vi "Destroy DataQ.vi"(6 "QueueName String (optional, otherwise \"\")":variant, 8 "error in (no error)":errorcluster, 9 "Select":T1, 10 "TaskName":string, 11 "DataQueues in":refnum<class "DataQueues.lvclass">) -> (0 "error out":errorcluster, 2 "TaskName out":string, 3 "DataQueues out":refnum<class "DataQueues.lvclass">)   [LabVIEW 2017, in "DataQueues.lvclass"]
doc: "Developed by Kevin Thompson\nkevin@thompsonengineering.net\n\nCopyright 2018-2020\nThompson Engineering, LLC"
uses:
  DataQueues.lvclass
  DataTypes/DataQ SelectType--enum.ctl
  DataQueues.lvclass/DataQueues.ctl
  DataTypes/DataQ Ref DictNode--cluster.ctl
  DataTypes/Analog DataSet SingleRow--QRef.ctl
  DataTypes/Analog DataSet SingleRow--cluster.ctl
  DataTypes/Analog DataSet MultiRow--QRef.ctl
  DataTypes/Analog DataSet MultiRow--cluster.ctl
  DataTypes/Analog DataSet MultiRow & ChanNames--QRef.ctl
  DataTypes/Analog DataSet MultiRow & ChanNames--cluster.ctl
  Accessors/Get QueueNames.vi
  Accessors/Get DataQ Dict.vi
  Accessors/Set QueueNames.vi
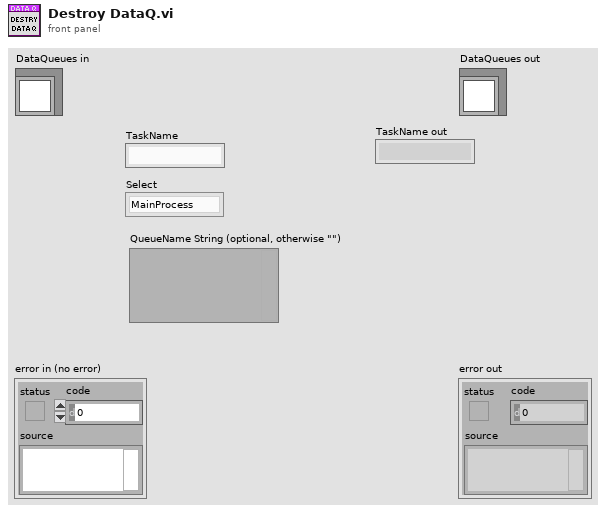
[diagram p1: front panel]
types:
  T1 = typedef "DataQueues.lvclass/DataQ SelectType--enum.ctl" = enum16{"MainProcess", "LogEngine", "LocalDAQThread"}
  T2 = typedef "DataQueues.lvclass/DataQ Ref DictNode--cluster.ctl" = cluster{"KeyName":string, "Type Name":string, "vDataQ Ref":variant}
  T3 = typedef "DataQueues.lvclass/Analog DataSet SingleRow--QRef.ctl" = refnum<queue>
  T4 = typedef "TD Dynamic CVT DVR--ref.ctl" = refnum<data-value>
  T5 = typedef "Type Descriptor Enumeration__ogtk.ctl" = enum8{"<Null>", "I8", "I16", "I32", "I64", "U8", "U16", "U32", "U64", "SGL", "DBL", "EXT", "CSG", "CDB", "CXT", "0x0F", "0x10", "0x11", "0x12", "0x13", "0x14", "Enum U8", "Enum U16", "Enum U32", "Enum U64", "SGL PQ", "DBL PQ", "EXT PQ", "CSG PQ", "CDB PQ", "CXT PQ", "0x1F", "0x20", "Boolean", "0x22", "0x23", "0x24", "0x25", "0x26", "0x27", "0x28", "0x29", "0x2A", "0x2B", "0x2C", "0x2D", "0x2E", "0x2F", "String", "0x31", "Path", "Pict", "0x34", "0x35", "0x36", "DAQ", "0x38", "0x39", "0x3A", "0x3B", "0x3C", "0x3D", "0x3E", "0x3F", "Array", "0x41", "0x42", "0x43", "0x44", "0x45", "0x46", "0x47", "0x48", "0x49", "0x4A", "0x4B", "0x4C", "0x4D", "0x4E", "0x4F", "Cluster", "0x51", "0x52", "Variant", "Waveform", "0x55", "0x56", "0x57", "0x58", "0x59", "0x5A", "0x5B", "0x5C", "0x5D", "0x5E", "0x5F", "0x60", "0x61", "0x62", "0x63", "0x64", "0x65", "0x66", "0x67", "0x68", "0x69", "0x6A", "0x6B", "0x6C", "0x6D", "0x6E", "0x6F", "Refnum"}
  T6 = typedef "DataQueues.lvclass/Analog DataSet MultiRow--QRef.ctl" = refnum<queue>
  T7 = typedef "DataQueues.lvclass/Analog DataSet MultiRow & ChanNames--QRef.ctl" = refnum<queue>
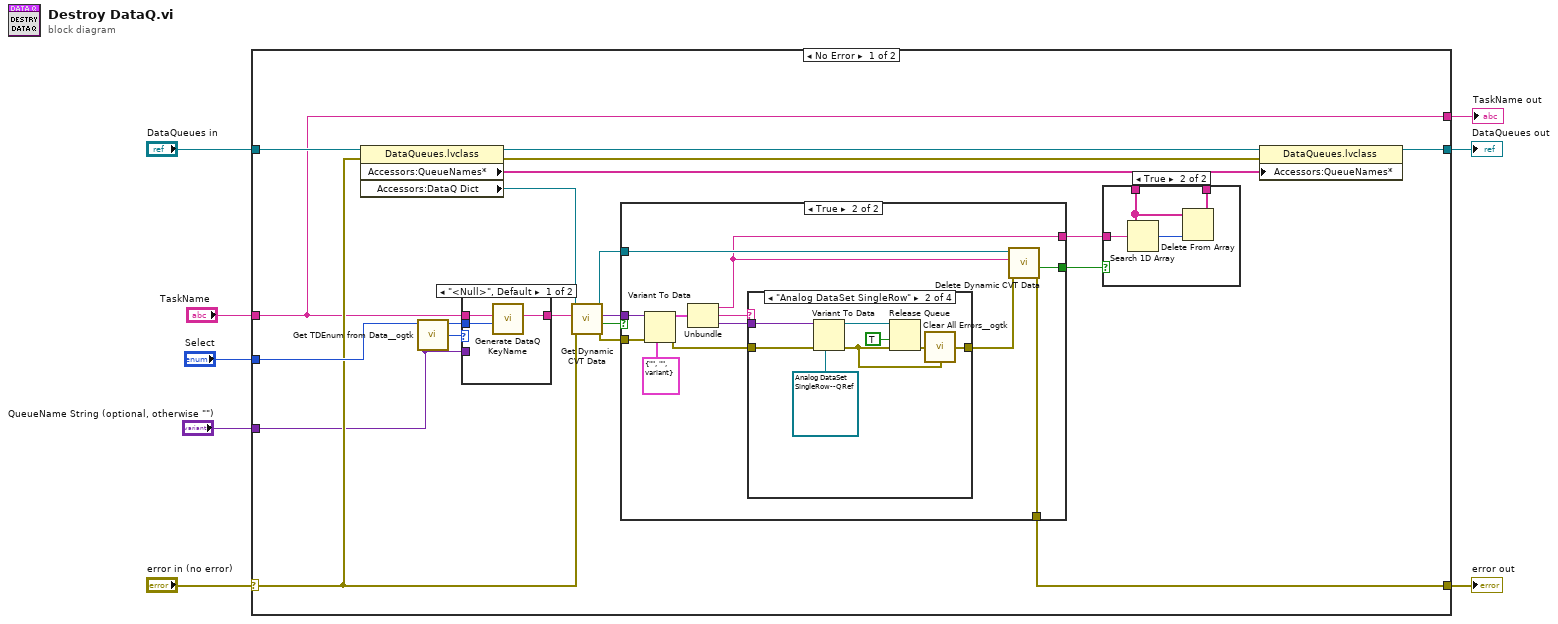
[diagram p0: block diagram]
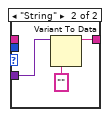
[diagram p2: hidden frame]
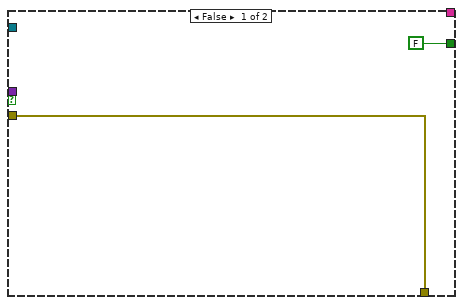
[diagram p3: hidden frame]
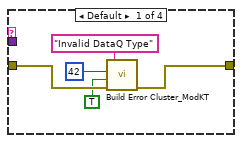
[diagram p4: hidden frame]
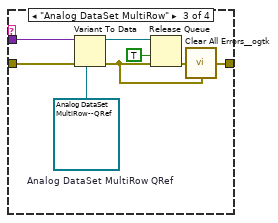
[diagram p5: hidden frame]
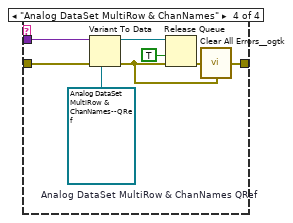
[diagram p6: hidden frame]
diagram:
  n1 = case shown="No Error" "error in (no error)" {
    selector: "error in (no error)" -> [w18 w85]
    tunnel: [w24 w85] -> w7
    tunnel: [w27 w84] -> w5
    tunnel: "DataQueues in" -> [w26 w84]
    tunnel: "TaskName" -> [w9 w83]
    tunnel: "Select" -> [w28 _]
    tunnel: "QueueName String (optional, otherwise \"\")" -> [w10 _]
    tunnel: [w9 w83] -> w1
    frame No Error {
      n2 = property class="DataQueues.lvclass"(reference=w26, error in=w18) -> (reference out=w25:refnum<class "DataQueues.lvclass">, error out=w23:errorcluster, "Accessors:QueueNames*"=w22:string[], "Accessors:DataQ Dict"=w19:T4)
      n3 = call <userlib>:"Get TDEnum from Data__ogtk.vi"("Data"=w10) -> ("Type Descriptor Enumeration"=w11:T5)  [unwired: 4 in]
      n4 = case shown="\"<Null>\", Default" w11 {
        tunnel: w9 -> [w31 _]
        tunnel: w28 -> [w30 _]
        tunnel: [w29 w34] -> w17
        tunnel: w10 -> [_ w33]
        frame "<Null>", Default {
          n5 = call "Generate DataQ KeyName.vi"("Select"=w30, "TaskName"=w31) -> ("DataQ KeyName"=w29:string)  [unwired: 9 in]
        }
        frame "String" {
          n6 = Variant To Data(type="", Variant=w33) -> (data=w34:string)  [unwired: 1 in, 1 out]
        }
      }
      n7 = call <vilib>:"Get Dynamic CVT Data.vi"("error in (no error)"=w18, "DataName"=w17, "dCVT DVR"=w19) -> ("error out"=w15:errorcluster, "found"=w12:bool, "value"=w16:variant, "dCVT DVR out"=w14:T4)  [unwired: 5 in]
      n8 = case shown="True" w12 {
        tunnel: [w35 w48] -> w24
        tunnel: [FALSE ("found") w47] -> w20
        tunnel: w16 -> [_ w46]
        tunnel: w15 -> [w35 w45]
        tunnel: w14 -> [_ w39]
        tunnel: [_ w38] -> w13
        frame False {
        }
        frame True {
          n9 = Variant To Data(error in=w45, type=T2 {"KeyName"="", "Type Name"="", "vDataQ Ref"=variant} ("DataQ Ref DictNode"), Variant=w46) -> (data=w43:T2, error out=w41:errorcluster)
          n10 = Unbundle(w43) -> ("KeyName"=w38:string, "Type Name"=w40:string, "vDataQ Ref"=w42:variant)
          n11 = case shown="\"Analog DataSet SingleRow\"" w40 {
            tunnel: w42 -> [_ w61 w69 w77]
            tunnel: w41 -> [w53 w60 w68 w75]
            tunnel: [w52 w55 w63 w70] -> w37
            frame Default {
              n12 = call <vilib>:"Build Error Cluster_ModKT .vi"("Prepend String (\"\")"="Invalid DataQ Type" ("Prepend String (\"\")"), "code"=42, "error? (F)"=TRUE, "error in (no error)"=w53) -> ("error out"=w52:errorcluster)  [unwired: 3 in, 1 out]
            }
            frame "Analog DataSet SingleRow" {
              n13 = Variant To Data(error in=w60, type=T3 refnum ("Analog DataSet SingleRow QRef"), Variant=w61) -> (data=w59:T3, error out=w56:errorcluster)
              n14 = Release Queue(queue=w59, force destroy? (F)=TRUE, error in (no error)=w56) -> (error out=w57:errorcluster)  [unwired: 2 out]
              n15 = call <userlib>:"Clear All Errors__ogtk.vi"("Upsteam Error (optional)"=w56, "Error In"=w57) -> ("Error Out"=w55:errorcluster)  [unwired: 2 in]
            }
            frame "Analog DataSet MultiRow" {
              w62 = T6 refnum  # Analog DataSet MultiRow QRef
              n16 = Variant To Data(error in=w68, type=w62, Variant=w69) -> (data=w67:T6, error out=w64:errorcluster)
              n17 = Release Queue(queue=w67, force destroy? (F)=TRUE, error in (no error)=w64) -> (error out=w65:errorcluster)  [unwired: 2 out]
              n18 = call <userlib>:"Clear All Errors__ogtk.vi"("Upsteam Error (optional)"=w64, "Error In"=w65) -> ("Error Out"=w63:errorcluster)  [unwired: 2 in]
            }
            frame "Analog DataSet MultiRow & ChanNames" {
              w76 = T7 refnum  # Analog DataSet MultiRow & ChanNames QRef
              n19 = Variant To Data(error in=w75, type=w76, Variant=w77) -> (data=w74:T7, error out=w71:errorcluster)
              n20 = Release Queue(queue=w74, force destroy? (F)=TRUE, error in (no error)=w71) -> (error out=w72:errorcluster)  [unwired: 2 out]
              n21 = call <userlib>:"Clear All Errors__ogtk.vi"("Upsteam Error (optional)"=w71, "Error In"=w72) -> ("Error Out"=w70:errorcluster)  [unwired: 2 in]
            }
          }
          n22 = call <vilib>:"Delete Dynamic CVT Data.vi"("error in (no error)"=w37, "DataName"=w38, "dCVT DVR"=w39) -> ("error out"=w48:errorcluster, "found"=w47:bool)  [unwired: 6 in, 1 out]
        }
      }
      n23 = case shown="True" w20 {
        tunnel: w13 -> [_ w82]
        tunnel: w22 -> [w78 w81]
        tunnel: [w78 w79] -> w21
        frame False {
        }
        frame True {
          n24 = Search 1D Array(1D array=w81, element=w82) -> (index of element=w80:i32)  [unwired: 1 in]
          n25 = Delete From Array(array=w81, index=w80) -> (array with subset deleted=w79:string[])  [unwired: 1 in, 1 out]
        }
      }
      n26 = property class="DataQueues.lvclass"(reference=w25, error in=w23, "Accessors:QueueNames*"=w21) -> (reference out=w27:refnum<class "DataQueues.lvclass">)  [unwired: 1 out]
    }
    frame Error {
    }
  }
  "error out" <- w7
  "DataQueues out" <- w5
  "TaskName out" <- w1
